vi "Add Class.vi"(8 "error in (no error)":errorcluster, 10 "Class":refnum<class "Class.lvclass">, 11 "Package in":refnum<class "Package.lvclass">) -> (0 "error out":errorcluster, 3 "Package out":refnum<class "Package.lvclass">)   [LabVIEW 2017, in "Cobertura.lvlib" / "Package.lvclass"]
uses:
  Package.lvclass
  Class/Class.lvclass
  Package.lvclass/Package.ctl
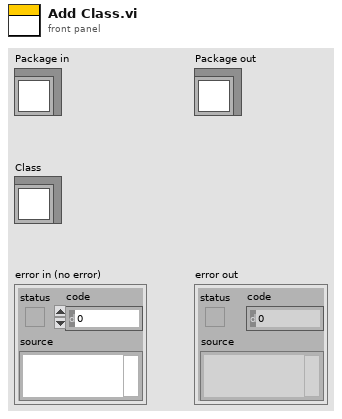
[diagram p1: front panel]
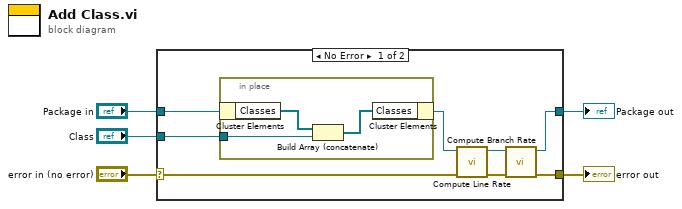
[diagram p0: block diagram]
diagram:
  n1 = case shown="No Error" "error in (no error)" {
    selector: "error in (no error)" -> [w13 w18]
    tunnel: [w9 w18] -> w4
    tunnel: [w6 w17] -> w2
    tunnel: "Package in" -> [w12 w17]
    tunnel: "Class" -> [w11 _]
    frame No Error {
      n2 = in-place {
        in-place-border: w11 -> [w14]
        n3 = in-place-cluster #1(w12) -> ("Classes"=w16:refnum<class "Class.lvclass">[])
        n4 = Build Array (concatenate)(w16, w14) -> (w15:refnum<class "Class.lvclass">[])
        n5 = in-place-cluster #1("Classes"=w15) -> (w8:refnum<class "Package.lvclass">)
      }
      n6 = call "Compute Line Rate.vi"("error in (no error)"=w13, "Package in"=w8) -> ("error out"=w10:errorcluster, "Package out"=w7:refnum<class "Package.lvclass">)  [unwired: 8 in]
      n7 = call "Compute Branch Rate.vi"("error in (no error)"=w10, "Package in"=w7) -> ("error out"=w9:errorcluster, "Package out"=w6:refnum<class "Package.lvclass">)  [unwired: 8 in]
    }
    frame Error {
    }
  }
  "error out" <- w4
  "Package out" <- w2
